vi "liq avg attri.vi"(11 "Dynamic Data":dynamicdata(waveform)) -> (3 "Signals Out":dynamicdata(waveform))   [LabVIEW 2016]
uses:
  <vilib>/express/express shared/transition.llb/Dynamic To Waveform Array.vi
  <vilib>/express/express signal manip/GetorSetDDTAttributes/Set DDT Attributes/SetT0.vi
  <vilib>/express/express shared/transition.llb/Waveform Array To Dynamic.vi
  <vilib>/express/express signal manip/GetorSetDDTAttributes/Set DDT Attributes/Set DDT Properties.xnode
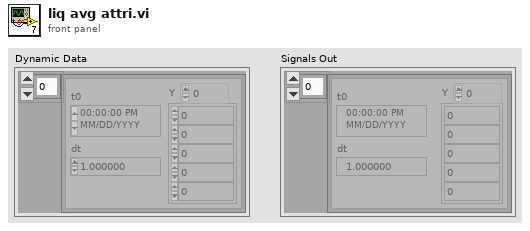
[diagram p1: front panel]
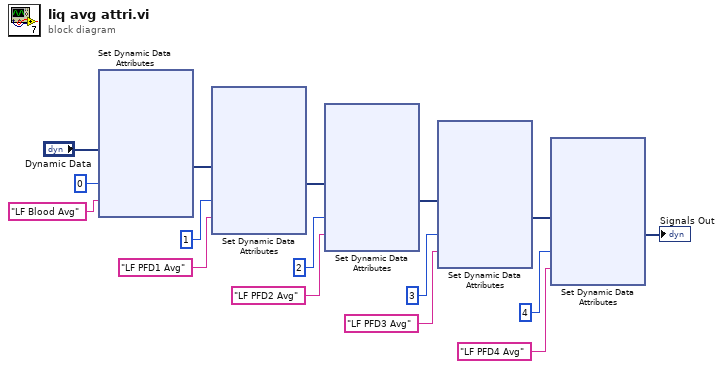
[diagram p0: block diagram]
diagram:
  n1 = xnode "Set Dynamic Data Attributes"("Signals In"="Dynamic Data", "Signal Index"=0, "Signal Name"="LF Blood Avg") -> ("Signals Out"=w4:dynamicdata)  [unwired: 1 in, 1 out]
  n2 = xnode "Set Dynamic Data Attributes"("Signals In"=w4, "Signal Index"=1, "Signal Name"="LF PFD1 Avg") -> ("Signals Out"=w7:dynamicdata)  [unwired: 1 in, 1 out]
  n3 = xnode "Set Dynamic Data Attributes"("Signals In"=w7, "Signal Index"=2, "Signal Name"="LF PFD2 Avg") -> ("Signals Out"=w10:dynamicdata)  [unwired: 1 in, 1 out]
  n4 = xnode "Set Dynamic Data Attributes"("Signals In"=w10, "Signal Index"=3, "Signal Name"="LF PFD3 Avg") -> ("Signals Out"=w13:dynamicdata)  [unwired: 1 in, 1 out]
  n5 = xnode "Set Dynamic Data Attributes"("Signals In"=w13, "Signal Index"=4, "Signal Name"="LF PFD4 Avg") -> ("Signals Out"=→"Signals Out":dynamicdata)  [unwired: 1 in, 1 out]
